vi "Default--constant.vi"(8 "error in":errorcluster, 11 "Generator in":refnum<class "Generador.lvclass">) -> (0 "error out":errorcluster, 3 "Generator out":refnum<class "Generador.lvclass">)   [LabVIEW 2020, in "FGen.lvlib" / "Generador.lvclass"]
uses:
  Generador.lvclass
  Generador.lvclass/Generador.ctl
  Set amplitude.vi
  Set frequency.vi
  Set offset.vi
  Set phase.vi
  Set sampling info.vi
  Set square wave duty cycle (%).vi
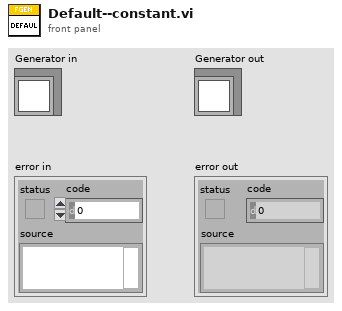
[diagram p1: front panel]
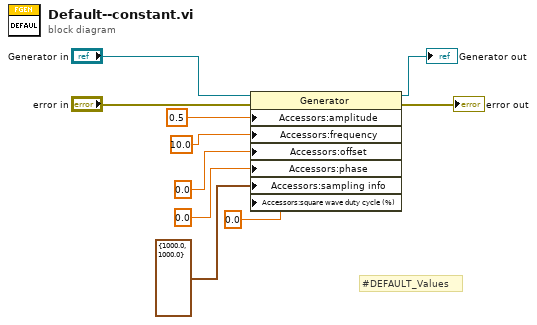
[diagram p0: block diagram]
diagram:
  # "#DEFAULT_Values"
  n1 = property class="Generator"(reference="Generator in", error in="error in", "Accessors:amplitude"=0.5 ("amplitude"), "Accessors:frequency"=10.0 ("frequency"), "Accessors:offset"=0.0 ("offset"), "Accessors:phase"=0.0 ("phase"), "Accessors:sampling info"=cluster{"Fs":dbl, "s":dbl} {"Fs"=1000.0, "s"=1000.0} ("sampling info"), "Accessors:square wave duty cycle (%)"=0.0 ("square wave duty cycle (%)")) -> (reference out=→"Generator out":refnum<class "Generador.lvclass">, error out=→"error out":errorcluster)
